vi "SV Append Data (1 Ch) (I32).vi"(7 "reset (F)":bool, 10 "maximum length (-1 = unlimited)":i32=-1, 11 "data in":i32=-2147483648) -> (3 "appended data":i32[](array[numeric]))   [LabVIEW 2017]
doc: "Use this VI to buffer data by appending input data to previously buffered data. Set the <B>maximum length</B> to set the buffered array size. The VI functions like a FIFO (First In, First Out) buffer, meaning that the oldest data is overwritten as new elements are added to the buffer. Wire data to the <B>data in</B> input to determine the polymorphic instance to use or manually select the instance."
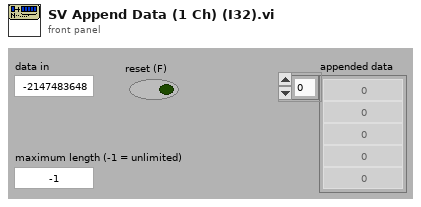
[diagram p1: front panel]
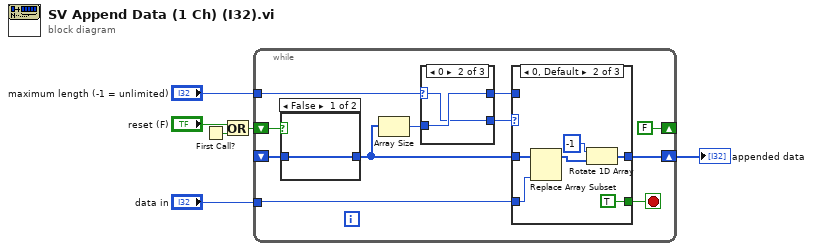
[diagram p0: block diagram]
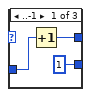
[diagram p2: hidden frame]
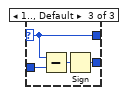
[diagram p3: hidden frame]
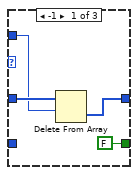
[diagram p4: hidden frame]
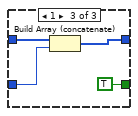
[diagram p5: hidden frame]
diagram:
  n1 = First Call?() -> (First Call?: T/F=w1:bool)
  n2 = Or(x="reset (F)", y=w1) -> (x .or. y?=w4:bool)
  n3 = while {
    tunnel: "data in" -> [w14]
    shift-right: [w13] -> w3
    shift-left: _ -> [w16]
    tunnel: "maximum length (-1 = unlimited)" -> [w7]
    shift-right: [FALSE] -> _
    shift-left: w4 -> [w17]
    stop <- w11 stop-if-true
    n4 = case shown="False" w17 {
      tunnel: [w41 _] -> w9
      tunnel: w16 -> [w41 _]
      frame False {
      }
      frame True {
      }
    }
    n5 = Array Size(array=w9) -> (size(s)=w8:i32)
    n6 = case shown="0" w7 {
      selector: w7 -> [_ w21 w23]
      tunnel: [1 w21 w25] -> w15
      tunnel: [w19 w22 w23] -> w10
      tunnel: w8 -> [w20 w22 w24]
      frame ..-1 {
        n7 = Increment(x=w20) -> (x+1=w19:i32)
      }
      frame 0 {
      }
      frame 1.., Default {
        n8 = Subtract(x=w23, y=w24) -> (x-y=w26:i32)
        n9 = Sign(1:w26) -> (0:w25:i32)
      }
    }
    n10 = case shown="0, Default" w15 {
      tunnel: w9 -> [w30 w36 w40]
      tunnel: w14 -> [_ w35 w39]
      tunnel: [w29 w33 w38] -> w13
      tunnel: w10 -> [w27 _ _]
      tunnel: [FALSE TRUE TRUE] -> w11
      frame -1 {
        n11 = Delete From Array(array=w30, length=w27) -> (deleted portion=w29:i32[])  [unwired: 1 in, 1 out]
      }
      frame 0, Default {
        n12 = Replace Array Subset(array=w36, new element=w35) -> (w34:i32[])  [unwired: 1 in]
        n13 = Rotate 1D Array(1:w34, 2:-1 ("n")) -> (0:w33:i32[])
      }
      frame 1 {
        n14 = Build Array (concatenate)(w40, w39) -> (w38:i32[])
      }
    }
  }
  "appended data" <- w3
